vi "rethinkdb_example_test.vi"() -> ()   [LabVIEW 2017]
uses:
  rethinkdb/RethinkDB.lvclass
panel:
  out "error out":errorcluster
  out "token out":u64 format="%016x"
  out "response":string
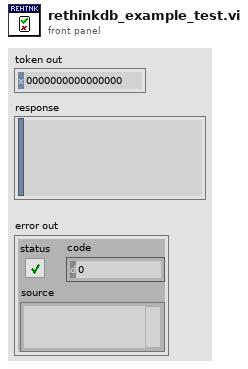
[diagram p1: front panel]
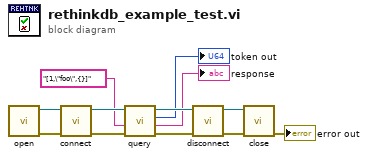
[diagram p0: block diagram]
diagram:
  n1 = call "open.vi"() -> ("error out"=w12:errorcluster, "rethinkdb out"=w11:refnum<class "RethinkDB.lvclass">)  [unwired: 10 in]
  n2 = call "connect.vi"("error in (no error)"=w12, "rethinkdb in"=w11) -> ("error out"=w8:errorcluster, "rethinkdb out"=w6:refnum<class "RethinkDB.lvclass">)  [unwired: 8 in]
  n3 = call "query.vi"("error in (no error)"=w8, "query"="[1,\"foo\",{}]", "rethinkdb in"=w6) -> ("error out"=w7:errorcluster, "response"=→"response":string, "token out"=→"token out":u64, "rethinkdb out"=w5:refnum<class "RethinkDB.lvclass">)  [unwired: 5 in]
  n4 = call "disconnect.vi"("error in (no error)"=w7, "rethinkdb in"=w5) -> ("error out"=w10:errorcluster, "rethinkdb out"=w9:refnum<class "RethinkDB.lvclass">)  [unwired: 8 in]
  n5 = call "close.vi"("error in (no error)"=w10, "rethinkdb in"=w9) -> ("error out"=→"error out":errorcluster)  [unwired: 9 in]
